vi "lockinSettings.vi"(6 "Error in (no error)":errorcluster, 9 "Application ref in":refnum<vi>) -> (0 "Error out":errorcluster, 2 "concatenated string":string, 3 "Application ref out":refnum<vi>)   [LabVIEW 2021]
uses:
  <userlib>/Nanonis Prog Interface V5/Nanonis Prog Interface.lvlib
panel:
  in  "Cluster 2":T1 {"Amplitude (mod. signal unit)" format="%#_6p"; "Frequency (Hz)" format="%#_6p"}
  out "Demod 2":T2
  out "Demod 1":T2
  in  "Cluster":T2 {"HP Filter Order" max=8 step=1; "LP Filter Order" max=8 step=1}
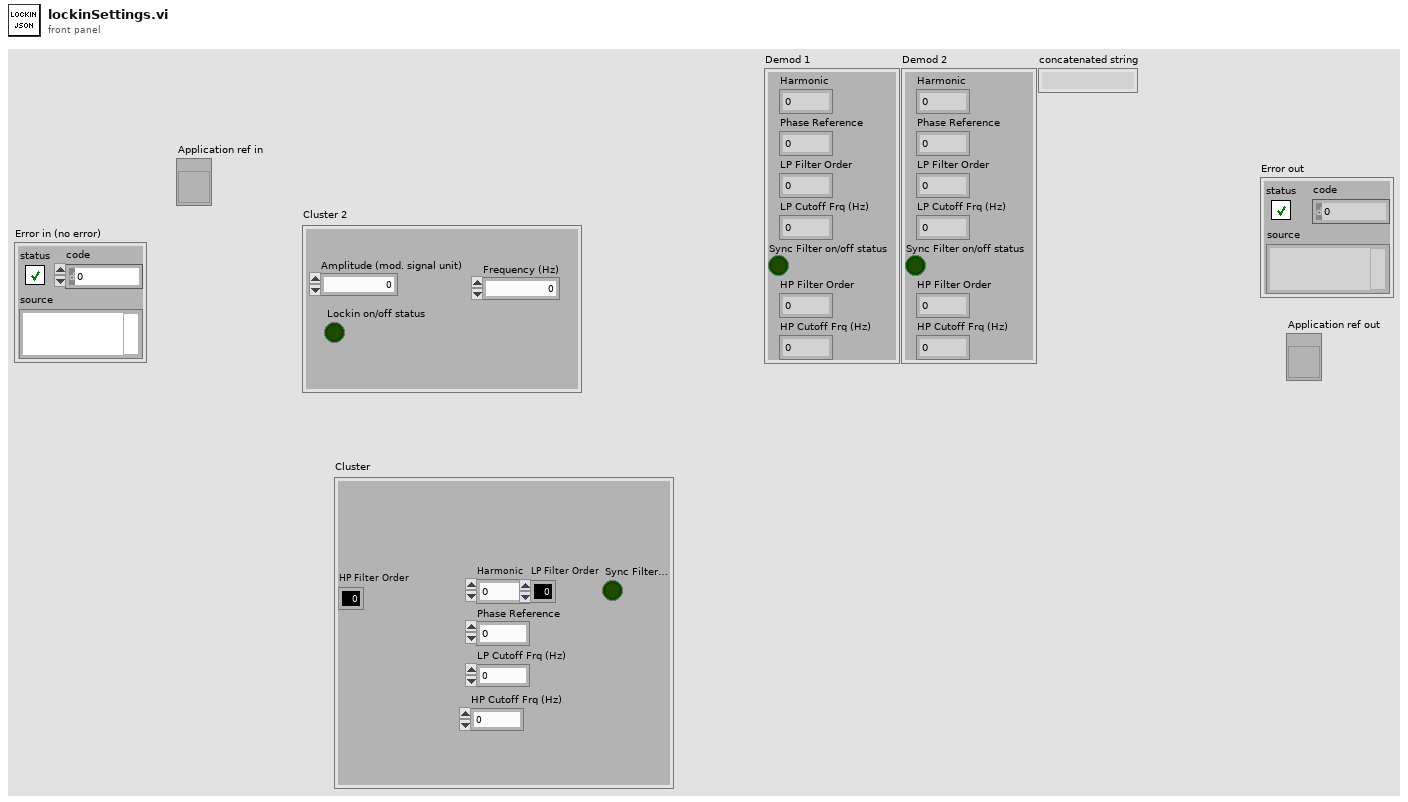
[diagram p1: front panel]
types:
  T1 = cluster{"Frequency (Hz)":dbl, "Amplitude (mod. signal unit)":sgl, "Lockin on/off status":bool}
  T2 = cluster{"Harmonic":u8, "Phase Reference":sgl, "LP Filter Order":u16, "LP Cutoff Frq (Hz)":sgl, "Sync Filter on/off status":bool, "HP Filter Order":u16, "HP Cutoff Frq (Hz)":sgl}
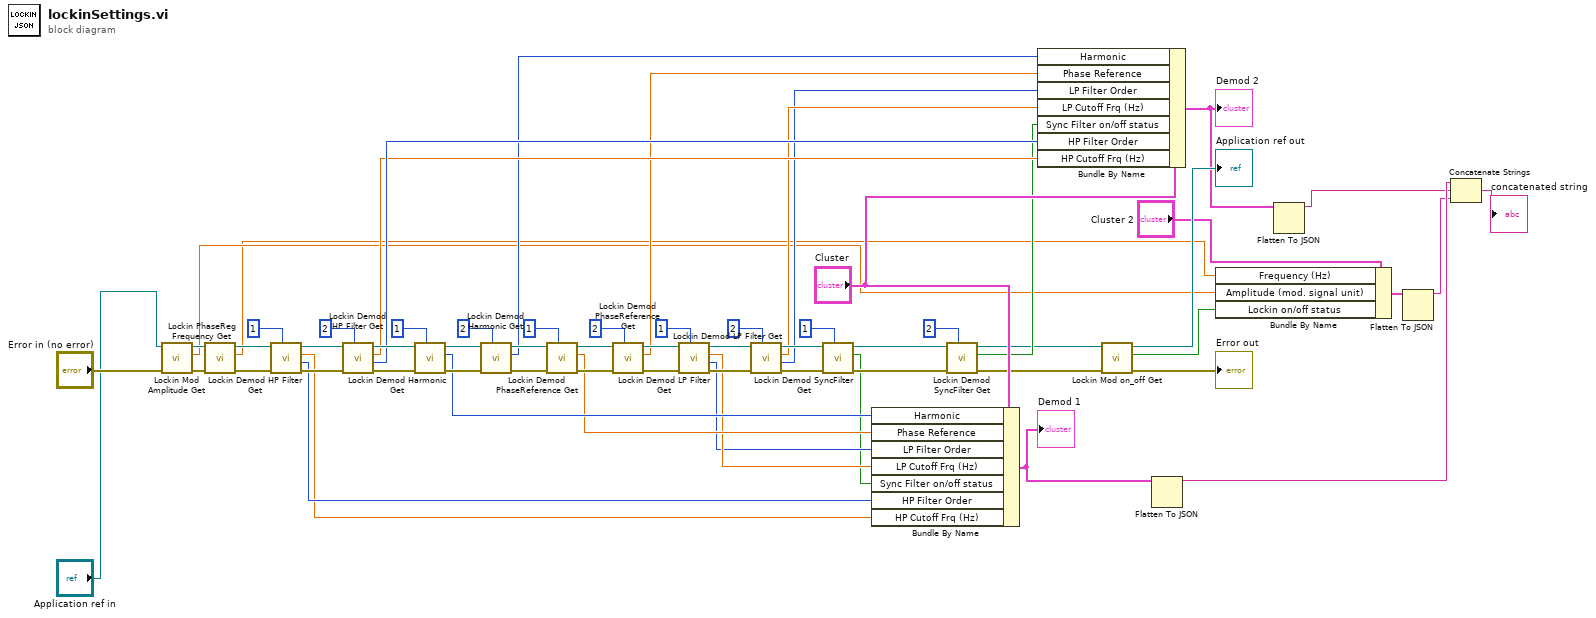
[diagram p0: block diagram]
diagram:
  n1 = call <userlib>:"Lockin Mod Amplitude Get.vi"("Error in (no error)"="Error in (no error)", "Application ref in"="Application ref in") -> ("Error out"=w64:errorcluster, "Amplitude (mod. signal unit)"=w11:sgl, "Application ref out"=w63:refnum<vi>)  [unwired: 7 in]
  n2 = call <userlib>:"Lockin PhaseReg Frequency Get.vi"("Error in (no error)"=w64, "Application ref in"=w63) -> ("Error out"=w62:errorcluster, "Frequency (Hz)"=w10:dbl, "Application ref out"=w61:refnum<vi>)  [unwired: 7 in]
  n3 = call <userlib>:"Lockin Demod HP Filter Get.vi"("Demodulator Index (1)"=1, "Error in (no error)"=w62, "Application ref in"=w61) -> ("Error out"=w59:errorcluster, "HP Filter Order"=w30:u16, "HP Cutoff Frq (Hz)"=w21:sgl, "Application ref out"=w60:refnum<vi>)  [unwired: 5 in]
  n4 = call <userlib>:"Lockin Demod HP Filter Get.vi"("Demodulator Index (1)"=2, "Error in (no error)"=w59, "Application ref in"=w60) -> ("Error out"=w58:errorcluster, "HP Filter Order"=w29:u16, "HP Cutoff Frq (Hz)"=w28:sgl, "Application ref out"=w57:refnum<vi>)  [unwired: 5 in]
  n5 = call <userlib>:"Lockin Demod Harmonic Get.vi"("Demodulator Index (1)"=1, "Error in (no error)"=w58, "Application ref in"=w57) -> ("Error out"=w55:errorcluster, "Harmonic"=w22:u8, "Application ref out"=w56:refnum<vi>)  [unwired: 6 in]
  n6 = call <userlib>:"Lockin Demod Harmonic Get.vi"("Demodulator Index (1)"=2, "Error in (no error)"=w55, "Application ref in"=w56) -> ("Error out"=w50:errorcluster, "Harmonic"=w27:u8, "Application ref out"=w49:refnum<vi>)  [unwired: 6 in]
  n7 = call <userlib>:"Lockin Demod PhaseReference Get.vi"("Demodulator Index (1)"=1, "Error in (no error)"=w50, "Application ref in"=w49) -> ("Error out"=w48:errorcluster, "Phase Reference"=w20:sgl, "Application ref out"=w47:refnum<vi>)  [unwired: 6 in]
  n8 = call <userlib>:"Lockin Demod PhaseReference Get.vi"("Demodulator Index (1)"=2, "Error in (no error)"=w48, "Application ref in"=w47) -> ("Error out"=w44:errorcluster, "Phase Reference"=w26:sgl, "Application ref out"=w43:refnum<vi>)  [unwired: 6 in]
  n9 = call <userlib>:"Lockin Demod LP Filter Get.vi"("Demodulator Index (1)"=1, "Error in (no error)"=w44, "Application ref in"=w43) -> ("Error out"=w42:errorcluster, "LP Filter Order"=w18:u16, "LP Cutoff Frq (Hz)"=w19:sgl, "Application ref out"=w41:refnum<vi>)  [unwired: 5 in]
  n10 = call <userlib>:"Lockin Demod LP Filter Get.vi"("Demodulator Index (1)"=2, "Error in (no error)"=w42, "Application ref in"=w41) -> ("Error out"=w38:errorcluster, "LP Filter Order"=w24:u16, "LP Cutoff Frq (Hz)"=w25:sgl, "Application ref out"=w37:refnum<vi>)  [unwired: 5 in]
  n11 = call <userlib>:"Lockin Demod SyncFilter Get.vi"("Demodulator Index (1)"=1, "Error in (no error)"=w38, "Application ref in"=w37) -> ("Error out"=w36:errorcluster, "Sync Filter on/off status"=w17:bool, "Application ref out"=w35:refnum<vi>)  [unwired: 6 in]
  n12 = Bundle By Name(cluster="Cluster", "Harmonic"=w22, "Phase Reference"=w20, "LP Filter Order"=w18, "LP Cutoff Frq (Hz)"=w19, "Sync Filter on/off status"=w17, "HP Filter Order"=w30, "HP Cutoff Frq (Hz)"=w21) -> (w5:T2)
  "Demod 1" <- w5
  n13 = call <userlib>:"Lockin Demod SyncFilter Get.vi"("Demodulator Index (1)"=2, "Error in (no error)"=w36, "Application ref in"=w35) -> ("Error out"=w14:errorcluster, "Sync Filter on/off status"=w23:bool, "Application ref out"=w16:refnum<vi>)  [unwired: 6 in]
  n14 = Bundle By Name(cluster="Cluster", "Harmonic"=w27, "Phase Reference"=w26, "LP Filter Order"=w24, "LP Cutoff Frq (Hz)"=w25, "Sync Filter on/off status"=w23, "HP Filter Order"=w29, "HP Cutoff Frq (Hz)"=w28) -> (w4:T2)
  "Demod 2" <- w4
  n15 = call <userlib>:"Lockin Mod on_off Get.vi"("Error in (no error)"=w14, "Application ref in"=w16) -> ("Error out"=→"Error out":errorcluster, "Lockin on/off status"=w9:bool, "Application ref out"=→"Application ref out":refnum<vi>)  [unwired: 7 in]
  n16 = Flatten To JSON(anything=w5) -> (JSON string=w3:string)  [unwired: 2 in, 1 out]
  n17 = Bundle By Name(cluster="Cluster 2", "Frequency (Hz)"=w10, "Amplitude (mod. signal unit)"=w11, "Lockin on/off status"=w9) -> (w8:T1)
  n18 = Flatten To JSON(anything=w4) -> (JSON string=w2:string)  [unwired: 2 in, 1 out]
  n19 = Flatten To JSON(anything=w8) -> (JSON string=w1:string)  [unwired: 2 in, 1 out]
  n20 = Concatenate Strings(w3, w2, w1) -> (→"concatenated string":string)
